vi "FILE EXISTS? v0.3.vi"(1 "Dir Path":path=path "/Data1Mac/Data", 2 "FILESPEC":string="test.001") -> (0 "?":bool=TRUE)   [LabVIEW 2019]
doc: "Checks whether specified file exists or not. Scott Hannahs, FBNML, Feb 1992"
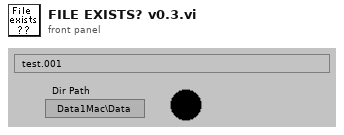
[diagram p1: front panel]
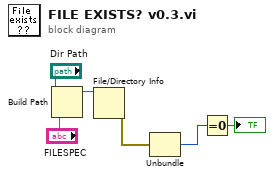
[diagram p0: block diagram]
diagram:
  n1 = Build Path(base path="Dir Path", name or relative path="FILESPEC") -> (appended path=w5:path)
  n2 = File/Directory Info(path=w5) -> (error out=w6:errorcluster)  [unwired: 1 in, 6 out]
  n3 = Unbundle(w6) -> ("code"=w1:i32)  [unwired: 2 out]
  n4 = Equal To 0?(x=w1) -> (x = 0?=→"?":bool)
